vi "niScope Error Message.vi"(0 "instrument handle":refnum<k15>, 5 "error code (0)":i32 format="%.0x", 11 "error in":errorcluster) -> (4 "instrument handle out":refnum<k15>, 8 "error message":string, 15 "error out":errorcluster)   [LabVIEW 2013]
doc: "Takes the error code returned by NI-SCOPE VIs and returns the interpretation as a user-readable string."
uses:
  niScope_32.dll
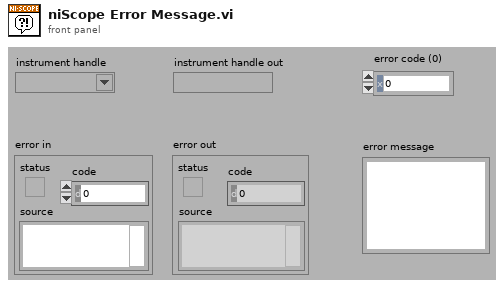
[diagram p1: front panel]
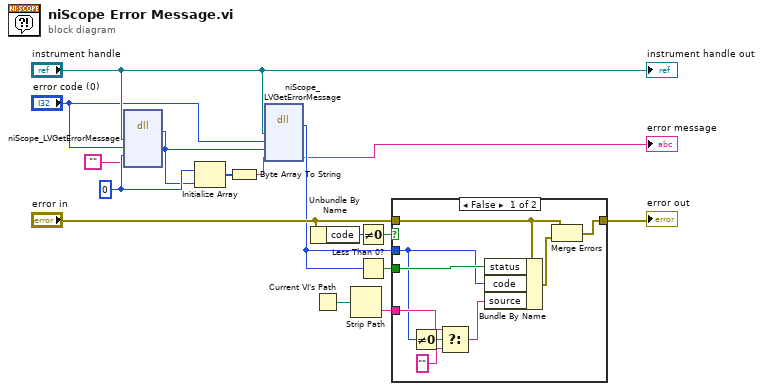
[diagram p0: block diagram]
diagram:
  w3 = u8 0
  n1 = dll-call lib="niScope_*.*" fn="niScope_LVGetErrorMessage" label="GetErrorMessage"("instrumentHandle"="instrument handle", "errorCode"="error code (0)", "bufferSize"=w3, "errorMessage"="") -> (w2:i32)  [unwired: 7 in, 2 out]
  n2 = Initialize Array(w3, w2) -> (w16:u8[])
  n3 = Byte Array To String(unsigned byte array=w16) -> (string=w8:string)
  n4 = dll-call lib="niScope_*.*" fn="niScope_LVGetErrorMessage" label="GetErrorMessage"("instrumentHandle"="instrument handle", "errorCode"="error code (0)", "bufferSize"=w2, "errorMessage"=w8) -> (w7:i32, "errorMessage"=→"error message":string)  [unwired: 6 in, 2 out]
  n5 = Unbundle By Name("error in") -> ("code"=w12:i32)
  n6 = Current VI's Path() -> (path=w11:path)
  n7 = Strip Path(path=w11) -> (name=w15:string)  [unwired: 1 out]
  n8 = Not Equal To 0?(x=w12) -> (x != 0?=w13:bool)
  n9 = Less Than 0?(x=w7) -> (x < 0?=w14:bool)
  n10 = case shown="False" w13 {
    tunnel: "error in" -> [w19 w26]
    tunnel: [w17 w26] -> w9
    tunnel: w14 -> [w23 _]
    tunnel: w15 -> [w22 _]
    tunnel: w7 -> [w20 _]
    frame False {
      n11 = Not Equal To 0?(x=w20) -> (x != 0?=w21:bool)
      n12 = Select(t=w22, s=w21, f="") -> (s? t:f=w24:string)
      n13 = Bundle By Name(cluster=w19, "status"=w23, "code"=w20, "source"=w24) -> (w18:errorcluster)
      n14 = Merge Errors(w19, w18) -> (w17:errorcluster)
    }
    frame True {
    }
  }
  "error out" <- w9
  "instrument handle out" <- "instrument handle"
